vi "Update.vi"(8 "error in (no error)":errorcluster, 10 "Message in":refnum<class "UpdateMessage.lvclass">, 11 "DAQMH121119OrcaFlash in":refnum<class "DAQOrcaFlash.lvclass">) -> (0 "error out":errorcluster, 3 "DAQMH121119OrcaFlash out":refnum<class "DAQOrcaFlash.lvclass">)   [LabVIEW 2012, in "DAQOrcaFlash.lvclass"]
doc: "The update method processes the command 'update'. \n\nThe command 'update' is used for receiving new values to be set to the private data of the class. This could be seen as a public set method for setting new parameters to the private class data."
uses:
  DAQOrcaFlash.lvclass
  <vilib>/Distrio/Murmex/UpdateMessage/UpdateMessage.lvclass
  DAQOrcaFlash.lvclass/DAQOrcaFlash.ctl
  merit_factor_type.ctl
  visualisation_line_cluster.ctl
  <vilib>/Distrio/Murmex/Murmex/Murmex.lvclass
panel:
  # "This method is called when the UPDATE\ntrigger is sent. \n\nOverride this method when your component needs to\nrespond to this trigger. \n\nCall parent for proper implementation"
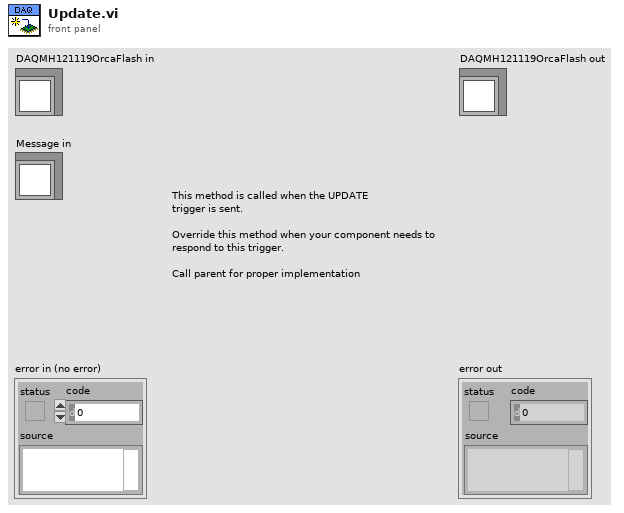
[diagram p1: front panel]
types:
  T1 = typedef "DAQOrcaFlash.lvclass/merit_factor_type.ctl" = enum16{"full frame intensity", "ROI beads", "Weber contrast", "Michelson contrast", "RMS contrast", "Line profile analysis", "ROI analysis", "FFT", "SNR", "5% brightest"}
  T2 = typedef "DAQOrcaFlash.lvclass/visualisation_line_cluster.ctl" = cluster{"direction":enum16{"horizontal", "vertical"}, "position":i32}
  T3 = typedef "IMAQ Image.ctl" = refnum<image>
  T4 = cluster{"Conversion Method":u32, "Minimum Value":i32, "Maximum Value":i32, "# Shifts":i32}
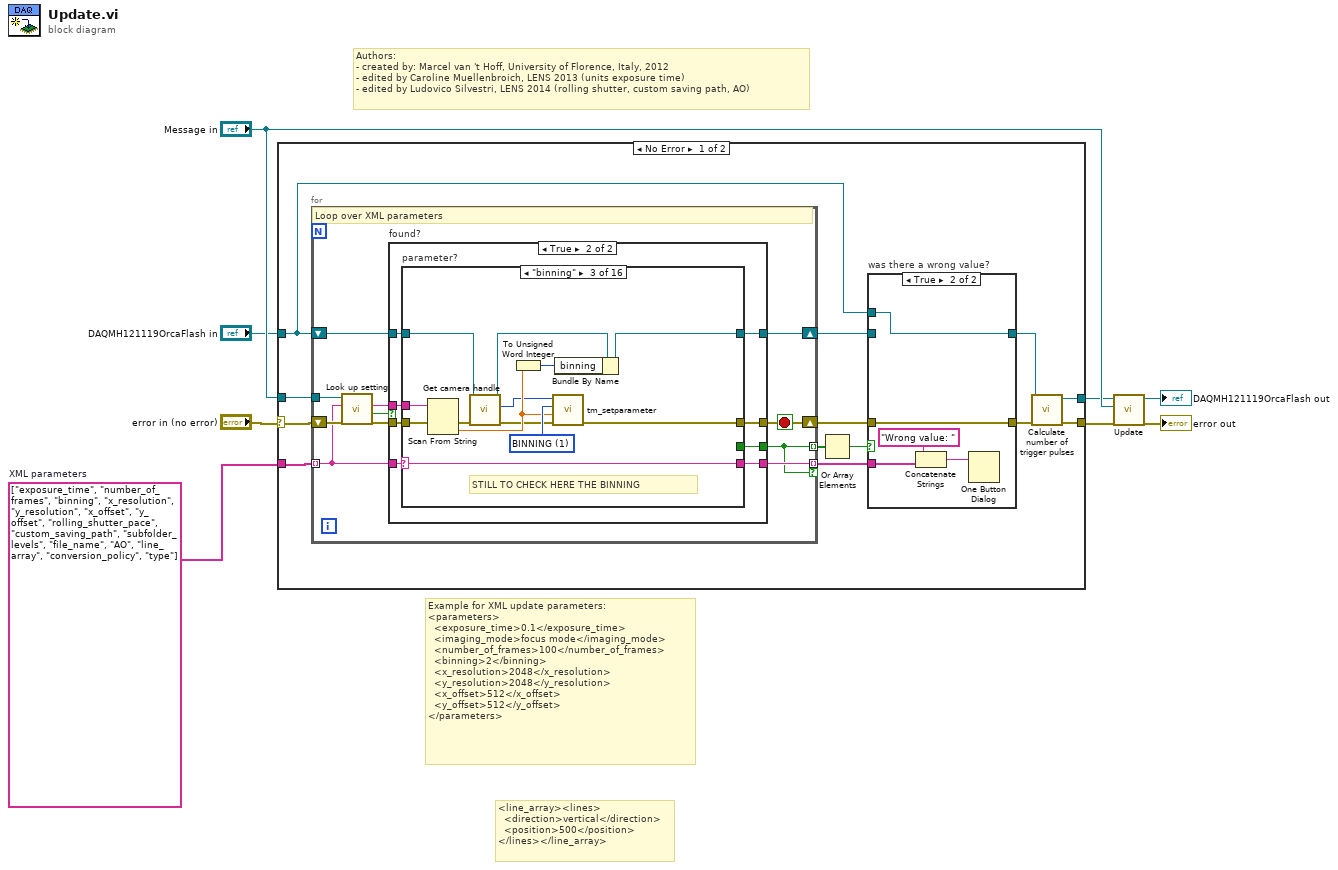
[diagram p0: block diagram]
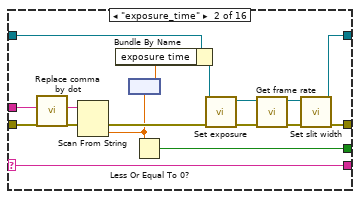
[diagram p5: hidden frame]
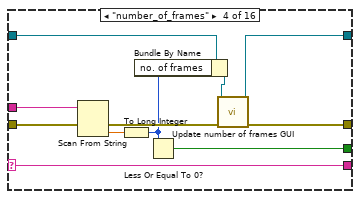
[diagram p6: hidden frame]
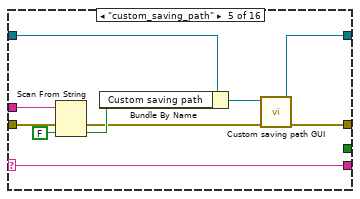
[diagram p7: hidden frame]
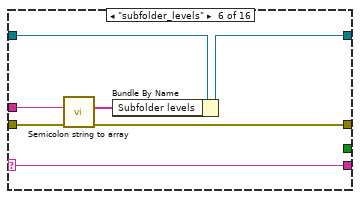
[diagram p8: hidden frame]
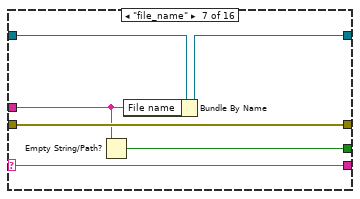
[diagram p9: hidden frame]
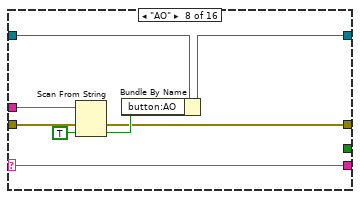
[diagram p10: hidden frame]
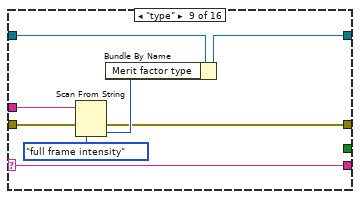
[diagram p11: hidden frame]
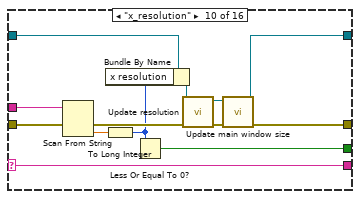
[diagram p12: hidden frame]
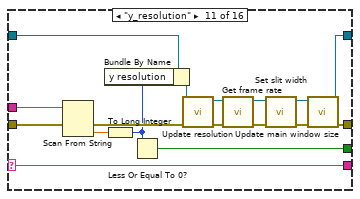
[diagram p13: hidden frame]
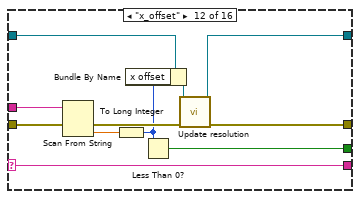
[diagram p14: hidden frame]
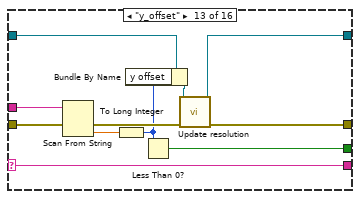
[diagram p15: hidden frame]
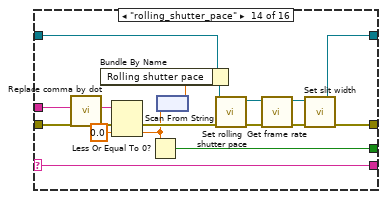
[diagram p16: hidden frame]
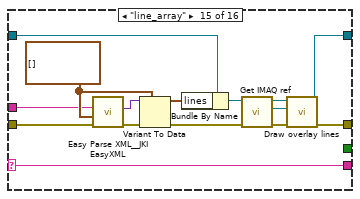
[diagram p17: hidden frame]
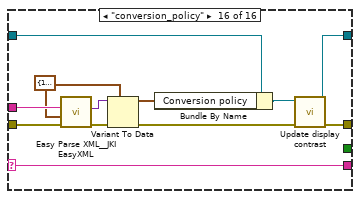
[diagram p18: hidden frame]
diagram:
  w8 = string[] ["exposure_time", "number_of_frames", "binning", "x_resolution", "y_resolution", "x_offset", "y_offset", "rolling_shutter_pace", "custom_saving_path", "subfolder_levels", "file_name", "AO", "line_array", "conversion_policy", "type"]  # XML parameters
  # "<line_array><lines>\n  <direction>vertical</direction>\n  <position>500</position>\n</lines></line_array>"
  # "Example for XML update parameters:\n<parameters>\n  <exposure_time>0.1</exposure_time>\n  <imaging_mode>focus mode</imaging_mode>\n  <number_of_frames>100</number_of_frames>\n  <binning>2</binning>\n  <x_resolution>2048</x_resolution>\n  <y_resolution>2048</y_resolution>\n  <x_offset>512</x_offset>\n  <y_offset>512</y_offset>\n</parameters>"
  # "Authors: \n- created by: Marcel van 't Hoff, University of Florence, Italy, 2012\n- edited by Caroline Muellenbroich, LENS 2013 (units exposure time)\n- edited by Ludovico Silvestri, LENS 2014 (rolling shutter, custom saving path, AO)"
  n1 = case shown="No Error" "error in (no error)" {
    selector: "error in (no error)" -> [w21 w230]
    tunnel: [w18 w230] -> w3
    tunnel: [w17 w229] -> w4
    tunnel: "DAQMH121119OrcaFlash in" -> [w14 w229]
    tunnel: "Message in" -> [w20 _]
    tunnel: w8 -> [w19 _]
    frame No Error {
      n2 = for "loop over parameters" {
        shift-right: [w37] -> w9
        shift-left: w21 -> [w35]
        shift-right: [w38] -> w12
        shift-left: w14 -> [w39]
        tunnel: w20 -> [w36]
        tunnel: w19 -> [w33] mode=indexing
        tunnel: [w29] -> w16 mode=indexing
        tunnel: [w30] -> w11 mode=indexing if=w29
        stop <- w37 stop-if-true
        # "Loop over XML parameters"
        n3 = call <vilib>:"Look up setting.vi"("error in (no error)"=w35, "tag name"=w33, "UpdateMessage in"=w36) -> ("error out"=w34:errorcluster, "found?"=w32:bool, "value"=w31:string)  [unwired: 5 in, 1 out]
        n4 = case "found?" shown="True" w32 {
          tunnel: w34 -> [w41 w50]
          tunnel: w31 -> [_ w49]
          tunnel: w33 -> [w40 w48]
          tunnel: w39 -> [w42 w47]
          tunnel: [w41 w46] -> w37
          tunnel: [w42 w45] -> w38
          tunnel: [_ w44] -> w29
          tunnel: [w40 w43] -> w30
          frame False {
          }
          frame True {
            # "XML parameter found?"
            n5 = case "parameter?" shown="\"binning\"" w48 {
              selector: w48 -> [w51 w54 w70 w85 w94 w104 w113 w117 w126 w133 w146 w163 w174 w185 w202 w217]
              tunnel: w50 -> [w52 w69 w82 w92 w100 w108 w114 w123 w132 w143 w160 w171 w182 w200 w212 w225]
              tunnel: w49 -> [_ w68 w81 w91 w101 w106 w112 w122 w131 w144 w161 w172 w183 w190 w213 w226]
              tunnel: w47 -> [w53 w59 w74 w93 w103 w110 w116 w121 w130 w145 w162 w173 w184 w201 w211 w224]
              tunnel: [w52 w63 w76 w88 w97 w107 w114 w118 w127 w139 w149 w167 w179 w195 w204 w221] -> w46
              tunnel: [w53 w62 w80 w86 w95 w109 w115 w119 w128 w137 w151 w166 w177 w194 w206 w220] -> w45
              tunnel: [_ w55 _ w83 _ _ w111 _ _ w134 w147 w164 w175 w186 _ _] -> w44
              tunnel: [w51 w54 w70 w85 w94 w104 w113 w117 w126 w133 w146 w163 w174 w185 w202 w217] -> w43
              frame Default {
              }
              frame "exposure_time" {
                n6 = call <vilib>:"Replace comma by dot.vi"("input string"=w68) -> ("result string"=w66:string)  [unwired: 10 in]
                n7 = Scan From String(input string=w66, error in=w69) -> (error out=w57:errorcluster, output 1=w56:dbl)  [unwired: 3 in, 2 out]
                n8 = node(w56) -> (w67:dbl[unit])
                n9 = Bundle By Name(cluster=w59, "exposure time"=w67) -> (w58:refnum<class "DAQOrcaFlash.lvclass">)
                n10 = Less Or Equal To 0?(x=w56) -> (x <= 0?=w55:bool)
                n11 = call-dynamic "Set exposure.vi"("error in (no error)"=w57, "DAQOrcaFlash in"=w58) -> ("error out"=w61:errorcluster, "DAQOrcaFlash out"=w60:refnum<class "DAQOrcaFlash.lvclass">)  [unwired: 8 in]
                n12 = call-dynamic "Get frame rate.vi"("error in (no error)"=w61, "DAQOrcaFlash in"=w60) -> ("error out"=w64:errorcluster, "DAQOrcaFlash out"=w65:refnum<class "DAQOrcaFlash.lvclass">)  [unwired: 8 in]
                n13 = call-dynamic "Set slit width.vi"("error in (no error)"=w64, "DAQOrcaFlash in"=w65) -> ("error out"=w63:errorcluster, "DAQOrcaFlash out"=w62:refnum<class "DAQOrcaFlash.lvclass">)  [unwired: 8 in]
              }
              frame "binning" {
                w79 = 1 items=["BINNING"=1, "BITS PER CHANNEL"=2, "ACTIVE VIEW INDEX"=3, "CCD MODE"=4, "SENSOR MODE"=5, "READOUT MODE"=6, "EXPOSURE TIME"=7, "CONTRAST GAIN"=8, "CONTRAST OFFSET"=9, "LIGHT MODE"=10, "SENSITIVITY"=11, "WHITE BALANCE"=12, "PHOTON IMAGING MODE"=13, "HIGH DYNAMIC RANGE MODE"=14, "TRIGGER SOURCE"=15, "TRIGGER ACTIVE"=16, "TRIGGER MODE"=17, "TRIGGER POLARITY"=18, "TRIGGER GLOBAL EXPOSURE"=19, "FIRST TRIGGER BEHAVIOR"=20, "TRIGGER TIMES"=21, "OUTPUT TRIGGER POLARITY"=22, "OUTPUT TRIGGER DELAY"=23, "OUTPUT TRIGGER PERIOD"=24, "TEMPERATURE"=25, "TEMPERATURE TARGET"=26, "SENSOR COOLER FAN"=27, "MECHANICAL SHUTTER"=28, "BACK FOCUS POSITION"=29, "FRAMEBUNDLE MODE"=30, "FRAMEBUNDLE NUMBER"=31] ("Parameter")
                # "STILL TO CHECK HERE THE BINNING"
                n14 = Scan From String(input string=w81, error in=w82) -> (error out=w77:errorcluster, output 1=w78:dbl)  [unwired: 3 in, 2 out]
                n15 = call "Get camera handle.vi"("error in (no error)"=w77, "DAQMH121119OrcaFlash in"=w74) -> ("error out"=w75:errorcluster, "cam handle"=w72:u32, "DAQMH121119OrcaFlash out"=w73:refnum<class "DAQOrcaFlash.lvclass">)  [unwired: 7 in]
                n16 = To Unsigned Word Integer(number=w78) -> (unsigned 16bit integer=w71:u16)
                n17 = call <userlib>:"tm_setparameter.vi"("error in (no error)"=w75, "Value in"=w78, "Parameter"=w79, "Handle in"=w72) -> ("error out"=w76:errorcluster)  [unwired: 6 in, 1 out]
                n18 = Bundle By Name(cluster=w73, "binning"=w71) -> (w80:refnum<class "DAQOrcaFlash.lvclass">)
              }
              frame "number_of_frames" {
                n19 = Scan From String(input string=w91, error in=w92) -> (error out=w89:errorcluster, output 1=w90:dbl)  [unwired: 3 in, 2 out]
                n20 = To Long Integer(number=w90) -> (32bit integer=w84:i32)
                n21 = Bundle By Name(cluster=w93, "no. of frames"=w84) -> (w87:refnum<class "DAQOrcaFlash.lvclass">)
                n22 = Less Or Equal To 0?(x=w84) -> (x <= 0?=w83:bool)
                n23 = call-dynamic "Update number of frames GUI.vi"("error in (no error)"=w89, "DAQOrcaFlash in"=w87) -> ("error out"=w88:errorcluster, "DAQOrcaFlash out"=w86:refnum<class "DAQOrcaFlash.lvclass">)  [unwired: 8 in]
              }
              frame "custom_saving_path" {
                n24 = Scan From String(input string=w101, error in=w100, default 1=FALSE) -> (error out=w98:errorcluster, output 1=w99:bool)  [unwired: 2 in, 2 out]
                n25 = Bundle By Name(cluster=w103, "Custom saving path"=w99) -> (w96:refnum<class "DAQOrcaFlash.lvclass">)
                n26 = call-dynamic "Custom saving path GUI.vi"("error in (no error)"=w98, "DAQOrcaFlash in"=w96) -> ("error out"=w97:errorcluster, "DAQOrcaFlash out"=w95:refnum<class "DAQOrcaFlash.lvclass">)  [unwired: 8 in]
              }
              frame "subfolder_levels" {
                n27 = call "Semicolon string to array.vi"("error in"=w108, "Semicolon string"=w106) -> ("error out"=w107:errorcluster, "String array"=w105:string[])  [unwired: 8 in]
                n28 = Bundle By Name(cluster=w110, "Subfolder levels"=w105) -> (w109:refnum<class "DAQOrcaFlash.lvclass">)
              }
              frame "file_name" {
                n29 = Empty String/Path?(string/path=w112) -> (empty?=w111:bool)
                n30 = Bundle By Name(cluster=w116, "File name"=w112) -> (w115:refnum<class "DAQOrcaFlash.lvclass">)
              }
              frame "AO" {
                n31 = Scan From String(input string=w122, error in=w123, default 1=TRUE) -> (error out=w118:errorcluster, output 1=w120:bool)  [unwired: 2 in, 2 out]
                n32 = Bundle By Name(cluster=w121, "button:AO"=w120) -> (w119:refnum<class "DAQOrcaFlash.lvclass">)
              }
              frame "type" {
                n33 = Scan From String(input string=w131, error in=w132, default 1=merit_factor_type."full frame intensity" ("settings.Merit factor type")) -> (error out=w127:errorcluster, output 1=w129:T1)  [unwired: 2 in, 2 out]
                n34 = Bundle By Name(cluster=w130, "Merit factor type"=w129) -> (w128:refnum<class "DAQOrcaFlash.lvclass">)
              }
              frame "x_resolution" {
                n35 = Scan From String(input string=w144, error in=w143) -> (error out=w136:errorcluster, output 1=w142:dbl)  [unwired: 3 in, 2 out]
                n36 = To Long Integer(number=w142) -> (32bit integer=w135:i32)
                n37 = Bundle By Name(cluster=w145, "x resolution"=w135) -> (w141:refnum<class "DAQOrcaFlash.lvclass">)
                n38 = Less Or Equal To 0?(x=w135) -> (x <= 0?=w134:bool)
                n39 = call "Update resolution.vi"("error in (no error)"=w136, "DAQMH121119OrcaFlash in"=w141) -> ("error out"=w140:errorcluster, "DAQMH121119OrcaFlash out"=w138:refnum<class "DAQOrcaFlash.lvclass">)  [unwired: 8 in]
                n40 = call "Update main window size.vi"("error in (no error)"=w140, "DAQOrcaFlash in"=w138) -> ("error out"=w139:errorcluster, "DAQOrcaFlash out"=w137:refnum<class "DAQOrcaFlash.lvclass">)  [unwired: 8 in]
              }
              frame "y_resolution" {
                n41 = Scan From String(input string=w161, error in=w160) -> (error out=w158:errorcluster, output 1=w159:dbl)  [unwired: 3 in, 2 out]
                n42 = To Long Integer(number=w159) -> (32bit integer=w148:i32)
                n43 = Bundle By Name(cluster=w162, "y resolution"=w148) -> (w157:refnum<class "DAQOrcaFlash.lvclass">)
                n44 = Less Or Equal To 0?(x=w148) -> (x <= 0?=w147:bool)
                n45 = call "Update resolution.vi"("error in (no error)"=w158, "DAQMH121119OrcaFlash in"=w157) -> ("error out"=w154:errorcluster, "DAQMH121119OrcaFlash out"=w153:refnum<class "DAQOrcaFlash.lvclass">)  [unwired: 8 in]
                n46 = call-dynamic "Get frame rate.vi"("error in (no error)"=w154, "DAQOrcaFlash in"=w153) -> ("error out"=w156:errorcluster, "DAQOrcaFlash out"=w155:refnum<class "DAQOrcaFlash.lvclass">)  [unwired: 8 in]
                n47 = call-dynamic "Set slit width.vi"("error in (no error)"=w156, "DAQOrcaFlash in"=w155) -> ("error out"=w150:errorcluster, "DAQOrcaFlash out"=w152:refnum<class "DAQOrcaFlash.lvclass">)  [unwired: 8 in]
                n48 = call "Update main window size.vi"("error in (no error)"=w150, "DAQOrcaFlash in"=w152) -> ("error out"=w149:errorcluster, "DAQOrcaFlash out"=w151:refnum<class "DAQOrcaFlash.lvclass">)  [unwired: 8 in]
              }
              frame "x_offset" {
                n49 = Scan From String(input string=w172, error in=w171) -> (error out=w169:errorcluster, output 1=w170:dbl)  [unwired: 3 in, 2 out]
                n50 = To Long Integer(number=w170) -> (32bit integer=w165:i32)
                n51 = Bundle By Name(cluster=w173, "x offset"=w165) -> (w168:refnum<class "DAQOrcaFlash.lvclass">)
                n52 = Less Than 0?(x=w165) -> (x < 0?=w164:bool)
                n53 = call "Update resolution.vi"("error in (no error)"=w169, "DAQMH121119OrcaFlash in"=w168) -> ("error out"=w167:errorcluster, "DAQMH121119OrcaFlash out"=w166:refnum<class "DAQOrcaFlash.lvclass">)  [unwired: 8 in]
              }
              frame "y_offset" {
                n54 = Scan From String(input string=w183, error in=w182) -> (error out=w180:errorcluster, output 1=w181:dbl)  [unwired: 3 in, 2 out]
                n55 = To Long Integer(number=w181) -> (32bit integer=w176:i32)
                n56 = Bundle By Name(cluster=w184, "y offset"=w176) -> (w178:refnum<class "DAQOrcaFlash.lvclass">)
                n57 = Less Than 0?(x=w176) -> (x < 0?=w175:bool)
                n58 = call "Update resolution.vi"("error in (no error)"=w180, "DAQMH121119OrcaFlash in"=w178) -> ("error out"=w179:errorcluster, "DAQMH121119OrcaFlash out"=w177:refnum<class "DAQOrcaFlash.lvclass">)  [unwired: 8 in]
              }
              frame "rolling_shutter_pace" {
                n59 = call <vilib>:"Replace comma by dot.vi"("input string"=w190) -> ("result string"=w189:string)  [unwired: 10 in]
                n60 = Scan From String(input string=w189, error in=w200, default 1=sgl 0.0 ("default value 1")) -> (error out=w199:errorcluster, output 1=w187:sgl)  [unwired: 2 in, 2 out]
                n61 = Less Or Equal To 0?(x=w187) -> (x <= 0?=w186:bool)
                n62 = node(w187) -> (w188:sgl[unit])
                n63 = Bundle By Name(cluster=w201, "Rolling shutter pace"=w188) -> (w198:refnum<class "DAQOrcaFlash.lvclass">)
                n64 = call-dynamic "Set rolling shutter pace.vi"("error in (no error)"=w199, "DAQOrcaFlash in"=w198) -> ("error out"=w197:errorcluster, "DAQOrcaFlash out"=w193:refnum<class "DAQOrcaFlash.lvclass">)  [unwired: 8 in]
                n65 = call-dynamic "Get frame rate.vi"("error in (no error)"=w197, "DAQOrcaFlash in"=w193) -> ("error out"=w196:errorcluster, "DAQOrcaFlash out"=w192:refnum<class "DAQOrcaFlash.lvclass">)  [unwired: 8 in]
                n66 = call-dynamic "Set slit width.vi"("error in (no error)"=w196, "DAQOrcaFlash in"=w192) -> ("error out"=w195:errorcluster, "DAQOrcaFlash out"=w194:refnum<class "DAQOrcaFlash.lvclass">)  [unwired: 8 in]
              }
              frame "line_array" {
                w215 = T2[] [] ("lines")
                n67 = call <vilib>:"Easy Parse XML__JKI EasyXML.vi"("error in (no error)"=w212, "LabVIEW Data (Type)"=w215, "XML String"=w213) -> ("error out"=w216:errorcluster, "LabVIEW Data"=w214:variant)  [unwired: 7 in]
                n68 = Variant To Data(error in=w216, type=w215, Variant=w214) -> (data=w210:T2[], error out=w209:errorcluster)
                n69 = Bundle By Name(cluster=w211, "lines"=w210) -> (w207:refnum<class "DAQOrcaFlash.lvclass">)
                n70 = call "Get IMAQ ref.vi"("error in (no error)"=w209, "DAQMH121119OrcaFlash in"=w207) -> ("error out"=w205:errorcluster, "IMAQ reference"=w203:T3, "DAQMH121119OrcaFlash out"=w208:refnum<class "DAQOrcaFlash.lvclass">)  [unwired: 7 in]
                n71 = call "Draw overlay lines.vi"("error in (no error)"=w205, "IMAQ reference"=w203, "DAQOrcaFlash in"=w208) -> ("error out"=w204:errorcluster, "DAQOrcaFlash out"=w206:refnum<class "DAQOrcaFlash.lvclass">)  [unwired: 6 in, 1 out]
              }
              frame "conversion_policy" {
                w218 = T4 {"Conversion Method"=10, "Minimum Value"=0, "Maximum Value"=1000, "# Shifts"=0} ("Conversion policy")
                n72 = call <vilib>:"Easy Parse XML__JKI EasyXML.vi"("error in (no error)"=w225, "LabVIEW Data (Type)"=w218, "XML String"=w226) -> ("error out"=w228:errorcluster, "LabVIEW Data"=w227:variant)  [unwired: 7 in]
                n73 = Variant To Data(error in=w228, type=w218, Variant=w227) -> (data=w223:T4, error out=w222:errorcluster)
                n74 = Bundle By Name(cluster=w224, "Conversion policy"=w223) -> (w219:refnum<class "DAQOrcaFlash.lvclass">)
                n75 = call-dynamic "Update display contrast.vi"("error in (no error)"=w222, "DAQOrcaFlash in"=w219) -> ("error out"=w221:errorcluster, "DAQOrcaFlash out"=w220:refnum<class "DAQOrcaFlash.lvclass">)  [unwired: 8 in]
              }
            }
          }
        }
      }
      n76 = Or Array Elements(Boolean array=w16) -> (logical OR=w15:bool)
      n77 = case "was there a wrong value?" shown="True" w15 {
        tunnel: w14 -> [_ w28]
        tunnel: [w23 w28] -> w13
        tunnel: w12 -> [w23 _]
        tunnel: w11 -> [_ w27]
        tunnel: [w22 w24] -> w10
        tunnel: w9 -> [w22 w24]
        frame False {
        }
        frame True {
          n78 = Concatenate Strings("Wrong value: " ("message"), w27) -> (w25:string)
          n79 = One Button Dialog(message=w25) -> ()  [unwired: 1 in, 1 out]
        }
      }
      n80 = call "Calculate number of trigger pulses.vi"("error in (no error)"=w10, "DAQOrcaFlash in"=w13) -> ("error out"=w18:errorcluster, "DAQOrcaFlash out"=w17:refnum<class "DAQOrcaFlash.lvclass">)  [unwired: 8 in]
    }
    frame Error {
    }
  }
  n81 = call-parent "Update.vi"("error in (no error)"=w3, "Message in"="Message in", "Murmex in"=w4) -> ("error out"=→"error out":errorcluster, "Murmex out"=→"DAQMH121119OrcaFlash out":refnum<class "DAQOrcaFlash.lvclass">)  [unwired: 7 in]
